vi "Correct Ascan.vi"(8 "error in":errorcluster caption="error out") -> (0 "error out":errorcluster caption="error in")   [LabVIEW 2015, in "Debug.lvlib"]
uses:
  Debug.lvlib
  Support/Filter Noise State.ctl
  <vilib>/Analysis/baseanly.llb/Mean (DBL).vi
  <vilib>/Utility/file.llb/Write Delimited Spreadsheet (DBL).vi
  <vilib>/Instr/_visa.llb/VISA Configure Serial Port (Instr).vi
  Sub VIs/DAQ/DAQ.lvlib
  Sub VIs/Digital Signal Processing/Digital Signal Processing.lvlib
  Sub VIs/Boimetry Processing/Boimetry Processing.lvlib
  <vilib>/Analysis/NI_AALBase.lvlib
  Sub VIs/Serial/Serial.lvlib
panel:
  out "进度条":u8(slide) scale=0.0..100.0
  out "DSP":dbl[](graph)
  out "Original Signal":dbl[](graph)
  in  "总长":dbl
  in  "步长":dbl
  in  "Sample Change":enum16{"1st", "2nd"}(ring)
  in  "DOUT":bool
  in  "计算":bool
  in  "采集":bool
  in  "停止按钮":bool
  out "距离点数":i32
  out "开始位置":i32
  out "状态栏":string
  # "Correct Ascan"
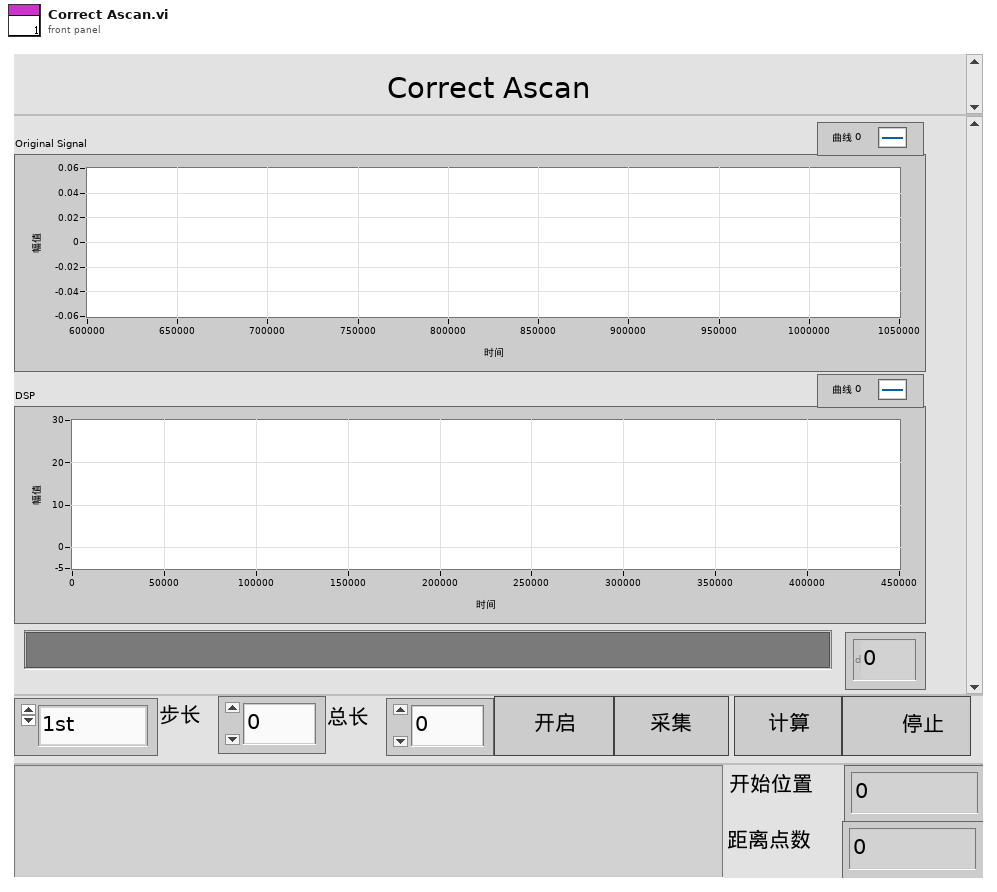
[diagram p1: front panel]
types:
  T1 = typedef "Debug.lvlib/Filter Noise State.ctl" = enum16{"Initialize", "Update Settings", "DOUT", "Sample", "Calculate", "Wait For Event", "Exit"}
  T2 = typedef "Digital Signal Processing.lvlib/DSP Configuration.ctl" = cluster{"Sampling Frequency":dbl, "filter type":T3, "RF Filter Low Frequency":dbl, "RF Filter High Frequency":dbl, "RF Filter Taps":i32, "window":T4, "RF window parameter":dbl, "filter type 2":T3, "Demodulated Filter Low Frequency":dbl, "Demodulated Filter HighFrequency":dbl, "Demodulated Filter Order":i32, "SPAN":i32, "Logarithmic Base":dbl, "Noise path":string, "Work position parameter":i32[]}
  T3 = typedef "NI_AALBase.lvlib/Filter Passband Type.ctl" = enum32{"Lowpass", "Highpass", "Bandpass", "Bandstop"}
  T4 = typedef "NI_AALPro.lvlib/windowTd.ctl" = u32
  T5 = typedef "Digital Signal Processing.lvlib/DSP Parameter.ctl" = cluster{"RF":cluster{"filter structure":enum32{"IIR 2nd Order", "IIR 4th Order"}, "Reverse Coefficients":dbl[], "Forward Coefficients":dbl[]}, "IIR Filter Cluster":cluster{"filter structure":enum32{"IIR 2nd Order", "IIR 4th Order"}, "Reverse Coefficients":dbl[], "Forward Coefficients":dbl[]}, "Noise Signal":dbl[], "SPAN":i32, "Logarithmic Base":dbl}
  T6 = cluster{"filter structure":enum32{"IIR 2nd Order", "IIR 4th Order"}, "Reverse Coefficients":dbl[], "Forward Coefficients":dbl[]}
  T7 = typedef "Boimetry Processing.lvlib/Biometry Configuration.ctl" = cluster{"Interference Width":i32, "Interference Threshold":dbl, "Cornea Len Division":i32, "Correction Data 1st Path":string, "1st_Start_Position":dbl, "Correction Data 2nd Path":string, "2nd_Start_Position":dbl, "Index Corneal":dbl, "Index Water":dbl, "Index Len":dbl, "Working Position":cluster{"FirstStart":i32, "FirstEnd":i32, "SecondStart":i32, "SecondEnd":i32}}
  T8 = cluster{"FirstStart":i32, "FirstEnd":i32, "SecondStart":i32, "SecondEnd":i32}
  T9 = typedef "DAQ.lvlib/DAQ Configuration.ctl" = cluster{"hDevice":i32, "DevNum":u8, "Configuration Parameter":i32[], "READ_MAX_LEN":i32, "DO":bool[]}
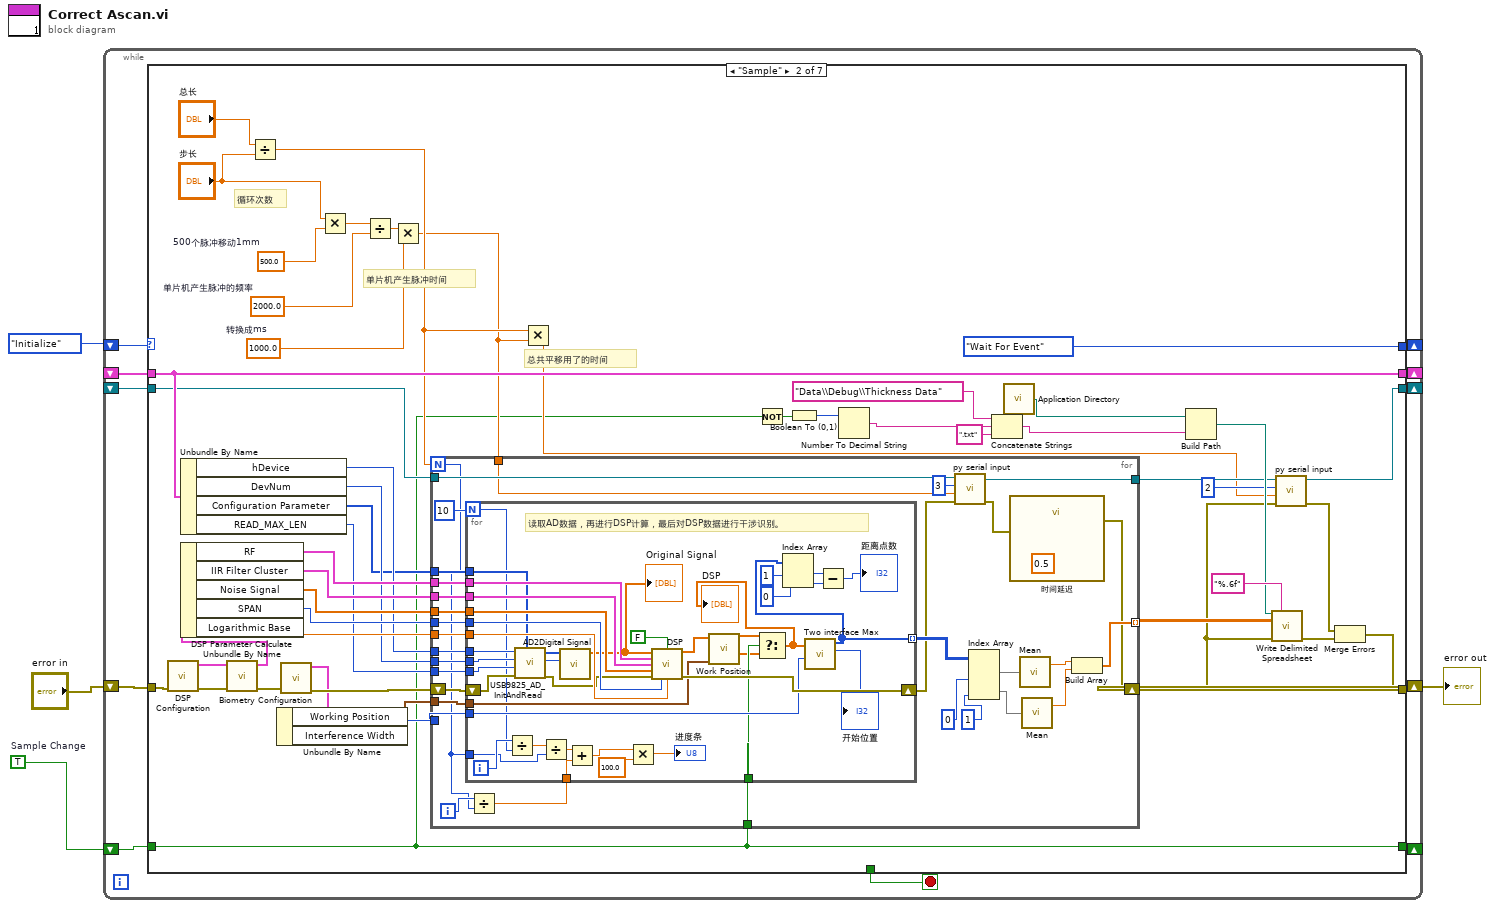
[diagram p0: block diagram]
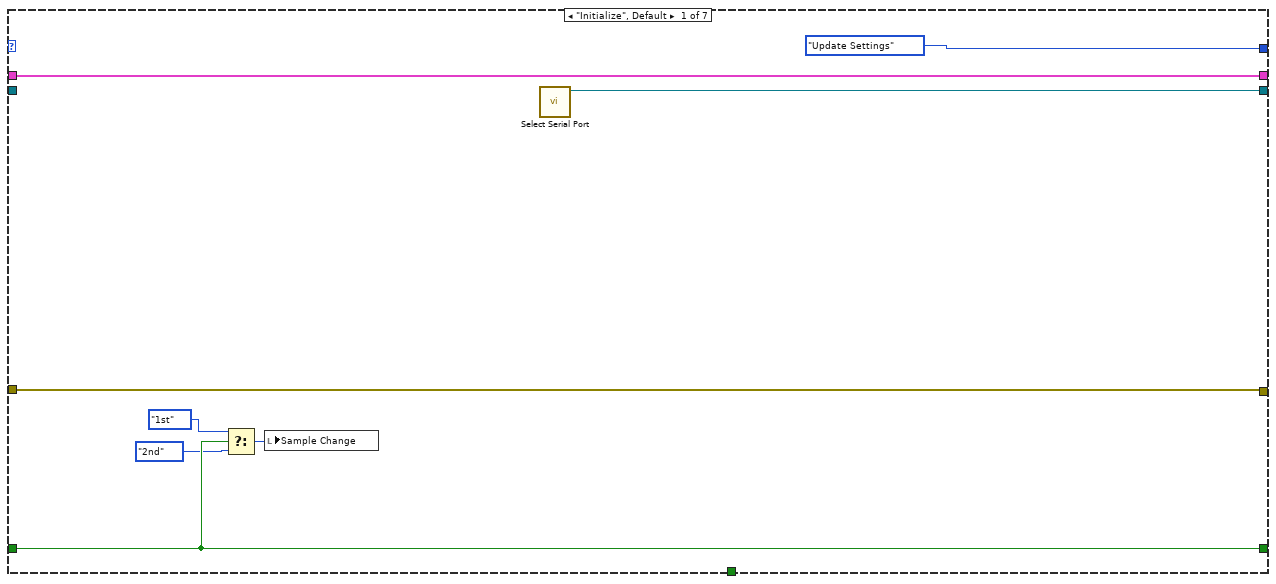
[diagram p2: hidden frame]
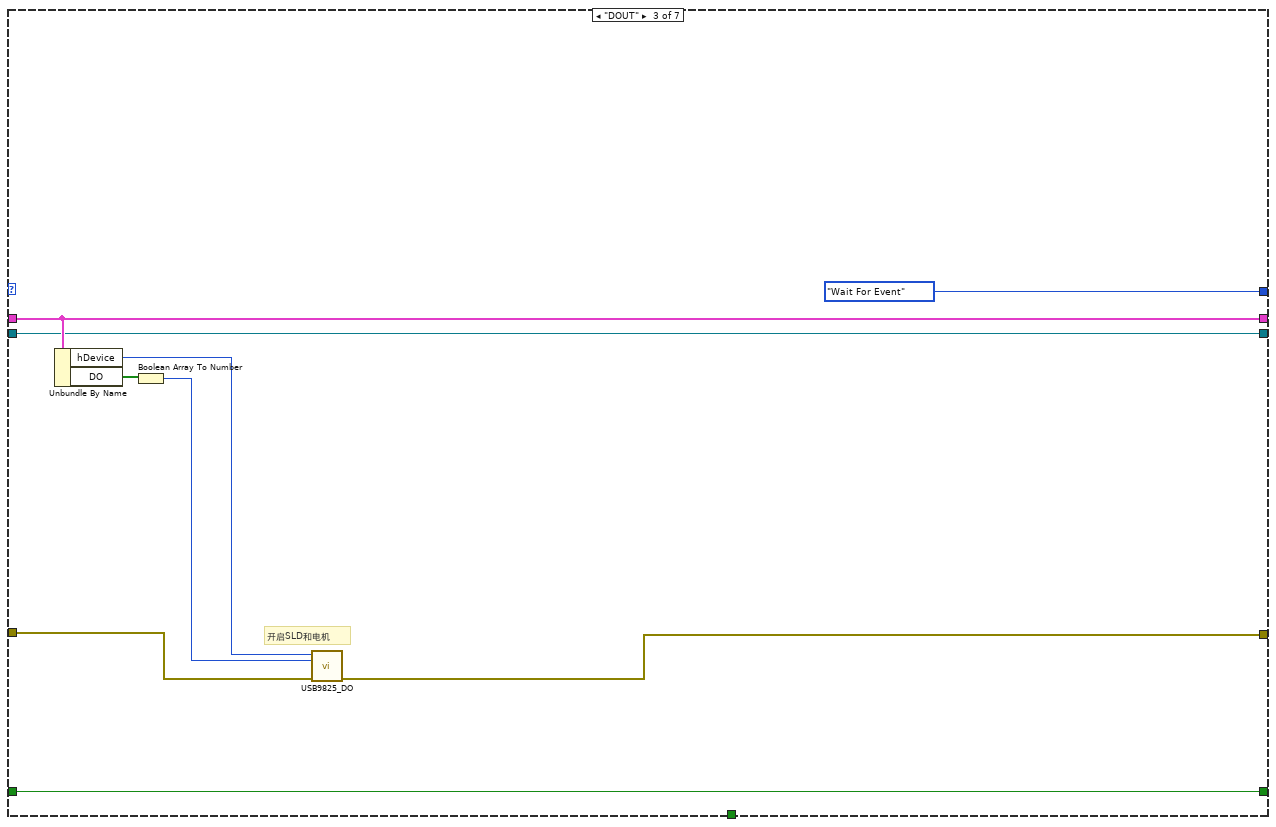
[diagram p3: hidden frame]
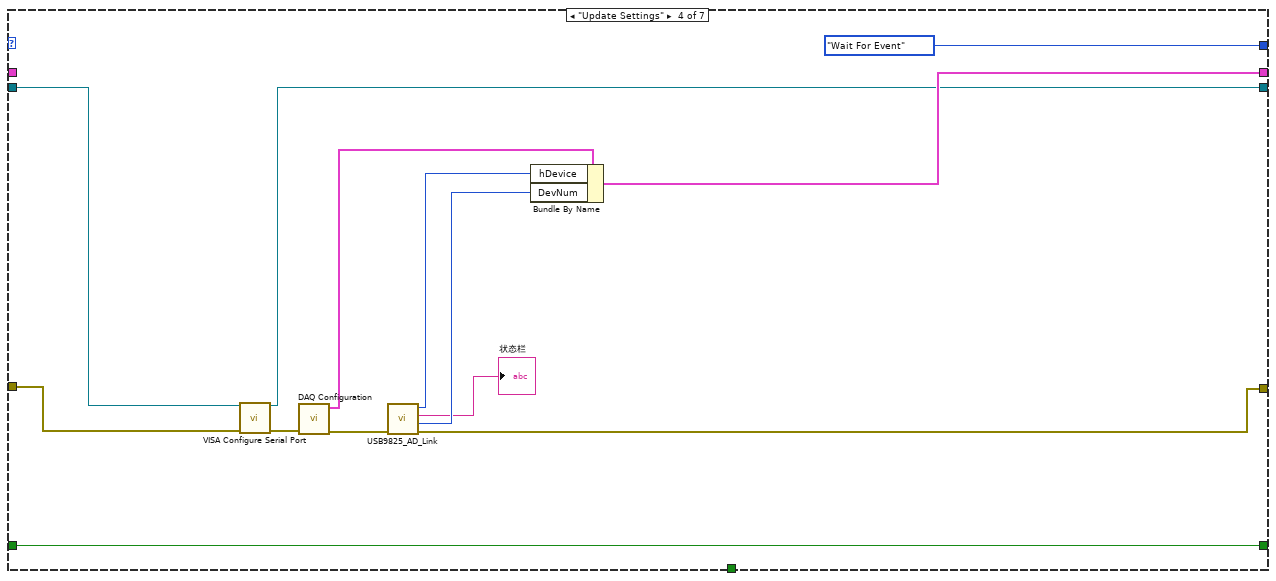
[diagram p4: hidden frame]
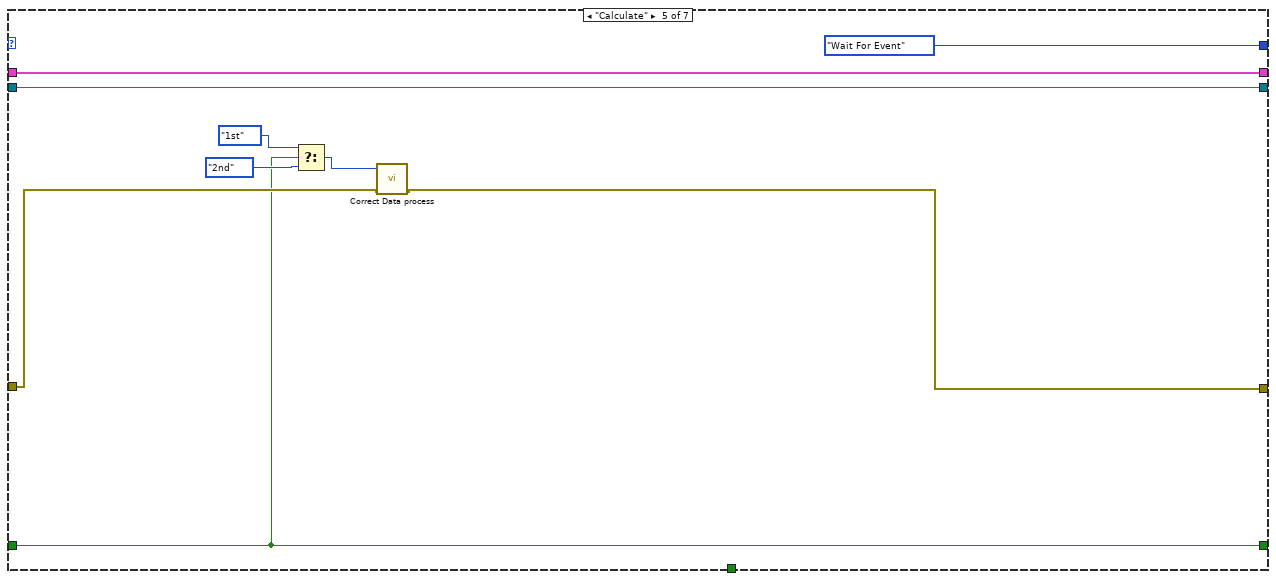
[diagram p5: hidden frame]
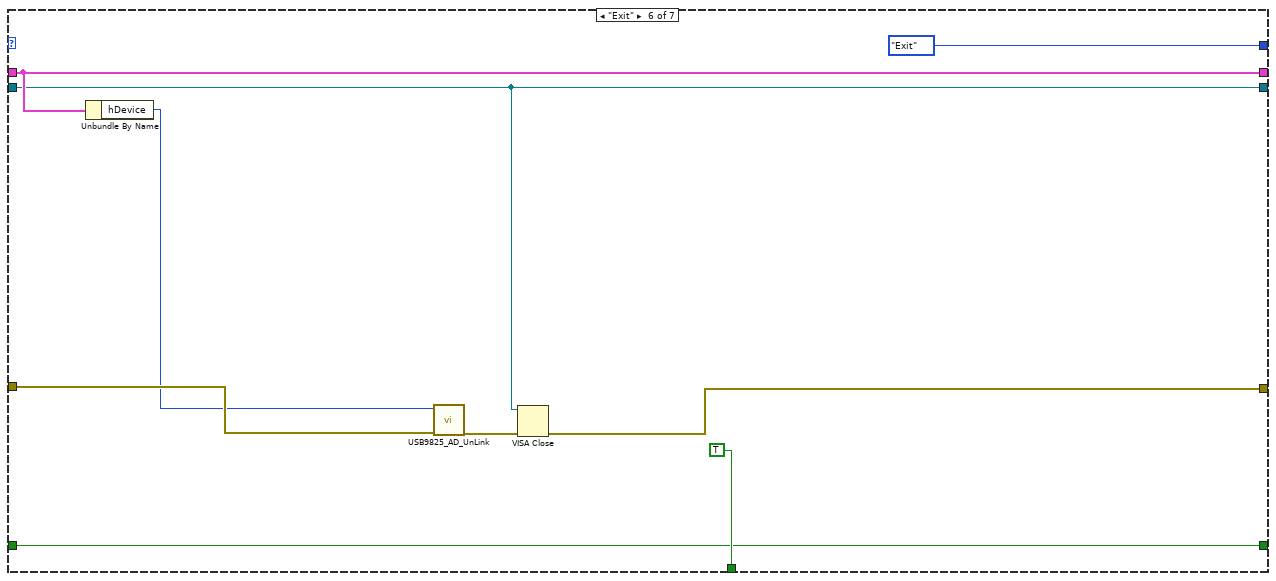
[diagram p6: hidden frame]
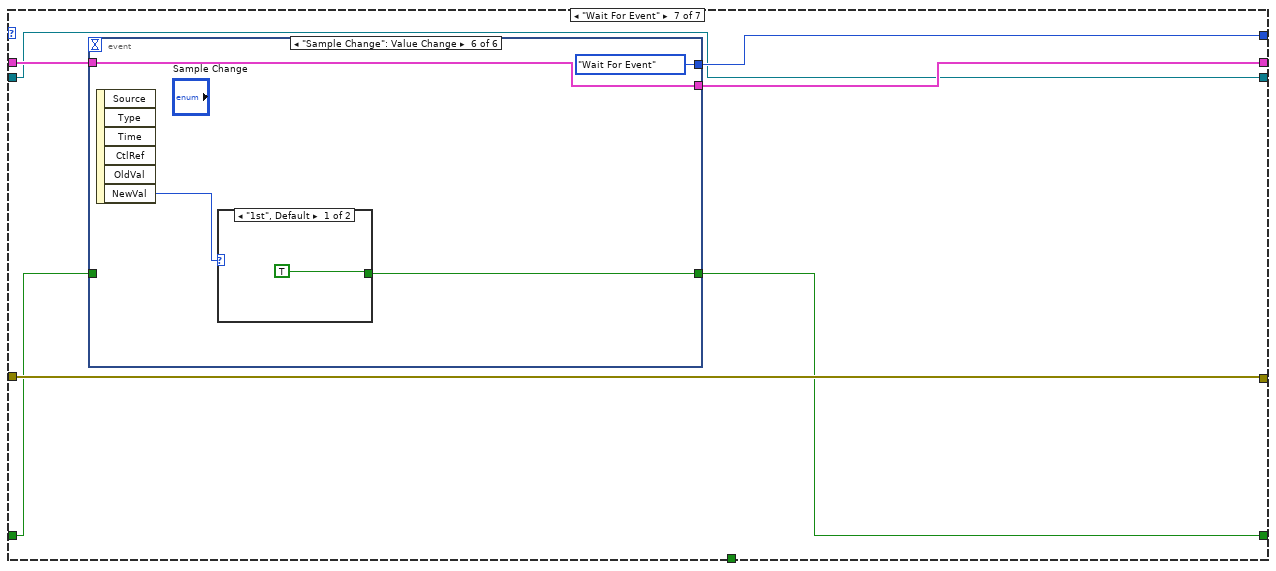
[diagram p7: hidden frame]
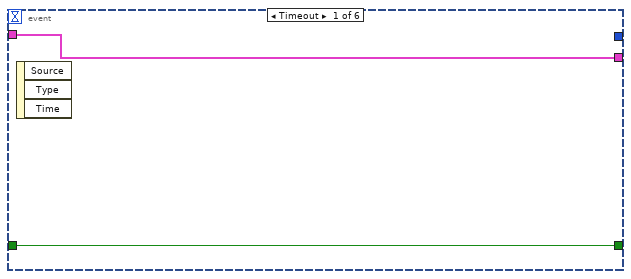
[diagram p8: hidden frame]
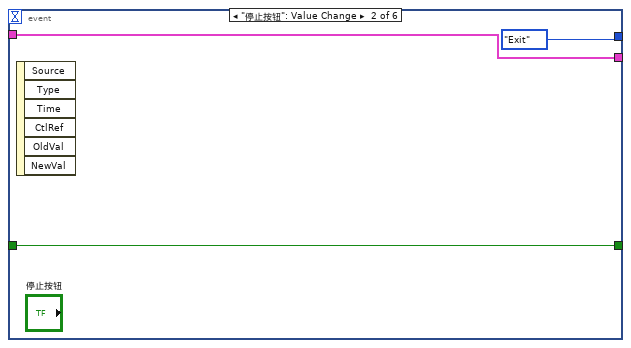
[diagram p9: hidden frame]
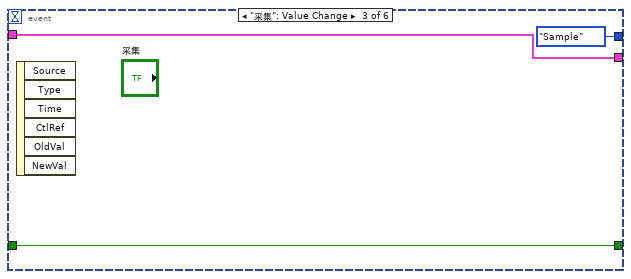
[diagram p10: hidden frame]
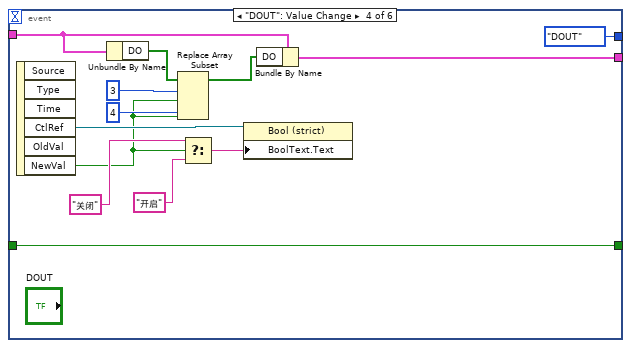
[diagram p11: hidden frame]
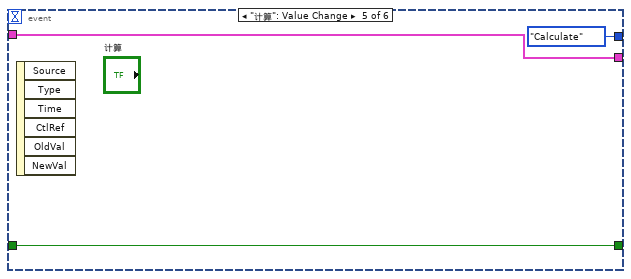
[diagram p12: hidden frame]
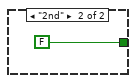
[diagram p13: hidden frame]
diagram:
  w1 = TRUE  # Sample Change
  n1 = while {
    shift-right: [w14] -> _
    shift-left: Filter_Noise_State."Initialize" ("Calculation Distance State") -> [w15]
    shift-right: [w12] -> w3
    shift-left: "error in" -> [w11]
    shift-right: [w10] -> _
    shift-left: _ -> [w9]
    shift-right: [w7] -> _
    shift-left: w1 -> [w8]
    shift-right: [w6] -> _
    shift-left: _ -> [w5]
    stop <- w13 stop-if-true
    n2 = case shown="\"Sample\"" w15 {
      tunnel: [Filter_Noise_State."Update Settings" ("Calculation Distance State") Filter_Noise_State."Wait For Event" ("Calculation Distance State") Filter_Noise_State."Wait For Event" ("Calculation Distance State") Filter_Noise_State."Wait For Event" ("Calculation Distance State") Filter_Noise_State."Wait For Event" ("Calculation Distance State") Filter_Noise_State."Exit" ("Calculation Distance State") w191] -> w14
      tunnel: [_ _ _ _ _ TRUE _] -> w13
      tunnel: w11 -> [w23 w70 w152 w155 w172 w182 w190]
      tunnel: [w23 w30 w151 w164 w171 w177 w190] -> w12
      tunnel: [w21 w71 w150 w160 w174 w181 w188] -> w10
      tunnel: w9 -> [w21 w71 w150 _ w174 w181 w189]
      tunnel: w8 -> [w19 w24 w146 w158 w167 w179 w186]
      tunnel: [w19 w24 w146 w158 w167 w179 w187] -> w7
      tunnel: [w18 w29 w145 w156 w173 w176 w185] -> w6
      tunnel: w5 -> [_ w47 w145 w157 w173 w176 w185]
      frame "Initialize", Default {
        n3 = Select(t=enum16{"1st", "2nd"}."1st" ("f"), s=w19, f=enum16{"1st", "2nd"}."2nd" ("Sample Change")) -> (s? t:f=w20:enum16{"1st", "2nd"})
        n4 = local write "Sample Change"(w20) -> ()
        n5 = call "Select Serial Port.vi"() -> ("VISA资源名称 2"=w18:refnum<visa-resource-name>)  [unwired: 11 in]
      }
      frame "Sample" {
        w27 = 1000.0  # 转换成ms
        w38 = 2000.0  # 单片机产生脉冲的频率
        w40 = 500.0  # 500个脉冲移动1mm
        # "总共平移用了的时间"
        # "单片机产生脉冲时间"
        # "循环次数"
        n6 = call "DSP Configuration.vi"("error in (no error)"=w70) -> ("error out"=w69:errorcluster, "DSP Parameter Output"=w62:T2)  [unwired: 9 in]
        n7 = Unbundle By Name(w71) -> ("hDevice"=w46:i32, "DevNum"=w45:u8, "Configuration Parameter"=w43:i32[], "READ_MAX_LEN"=w44:i32)
        n8 = call "DSP Parameter Calculate.vi"("error in (no error)"=w69, "DSP Configuration"=w62) -> ("error out"=w61:errorcluster, "DSP Parameter"=w68:T5)  [unwired: 8 in]
        n9 = Unbundle By Name(w68) -> ("RF"=w67:T6, "IIR Filter Cluster"=w66:T6, "Noise Signal"=w63:dbl[], "SPAN"=w65:i32, "Logarithmic Base"=w64:dbl)
        n10 = Divide(x="总长", y="步长") -> (x/y=w34:dbl)
        n11 = call "Biometry Configuration.vi"("error in (no error)"=w61) -> ("error out"=w60:errorcluster, "Biometry Configuration"=w59:T7)  [unwired: 9 in]
        n12 = Unbundle By Name(w59) -> ("Working Position"=w58:T8, "Interference Width"=w57:i32)
        n13 = Multiply(x="步长", y=w40) -> (x*y=w39:dbl)
        n14 = Divide(x=w39, y=w38) -> (x/y=w28:dbl)
        n15 = Multiply(x=w28, y=w27) -> (x*y=w26:dbl)
        n16 = for {
          N: w34 -> [w74]
          tunnel: w67 -> [w105]
          tunnel: w66 -> [w104]
          tunnel: w65 -> [w103]
          tunnel: w64 -> [w102]
          tunnel: w63 -> [w100]
          tunnel: w58 -> [w98]
          tunnel: w57 -> [w97]
          tunnel: w24 -> [w96]
          shift-right: [w77] -> w35
          shift-left: w60 -> [w99]
          tunnel: [w88] -> w56 mode=indexing
          tunnel: w47 -> [w86]
          tunnel: w46 -> [w85]
          tunnel: w45 -> [w84]
          tunnel: w44 -> [w83]
          tunnel: w43 -> [w82]
          tunnel: w26 -> [w81]
          tunnel: [w79] -> w37
          i -> [w75]
          n17 = Divide(x=w75, y=w74) -> (x/y=w73:dbl)
          n18 = for {
            N: 10 -> [w116]
            shift-right: [w144] -> w87
            shift-left: w99 -> [w139]
            tunnel: w105 -> [w143]
            tunnel: w104 -> [w142]
            tunnel: w103 -> [w141]
            tunnel: w102 -> [w140]
            tunnel: w100 -> [w135]
            tunnel: w98 -> [w132]
            tunnel: w97 -> [w131]
            tunnel: w96 -> [w130]
            tunnel: [w124] -> w95 mode=indexing
            tunnel: w85 -> [w129]
            tunnel: w84 -> [w128]
            tunnel: w83 -> [w127]
            tunnel: w82 -> [w126]
            tunnel: w74 -> [w114]
            tunnel: w73 -> [w111]
            i -> [w117]
            # "读取AD数据，再进行DSP计算，最后对DSP数据进行干涉识别。"
            n19 = Divide(x=w117, y=w116) -> (x/y=w115:dbl)
            n20 = call "USB9825_AD_InitAndRead.vi"("Configuration Parameter"=w126, "错误输入（无错误）"=w139, "READ_MAX_LEN"=w127, "DevNum"=w128, "hDevice"=w129) -> ("错误输出"=w136:errorcluster, "通道数"=w137:i32, "AD"=w138:i16[])  [unwired: 3 in, 1 out]
            n21 = Divide(x=w115, y=w114) -> (x/y=w112:dbl)
            n22 = call "AD2Digital Signal.vi"("通道数"=w137, "AD"=w138) -> ("CH1"=w133:dbl[])  [unwired: 8 in, 1 out]
            "Original Signal" <- w133
            n23 = Add(x=w112, y=w111) -> (x+y=w110:dbl)
            n24 = Multiply(x=w110, y=100.0) -> (x*y=→"进度条":dbl)
            n25 = call "DSP.vi"("Input Signal"=w133, "Minus Noise(F : Don't)"=FALSE ("Smooth(F : Don't)"), "RF"=w143, "IIR Filter Cluster"=w142, "Noise Signal"=w135, "error in (no error)"=w136, "SPAN"=w141, "Logarithmic Base"=w140) -> ("DSP signal"=w118:dbl[], "error out"=w144:errorcluster)  [unwired: 6 in]
            n26 = call "Work Position.vi"("Working Position"=w132, "S"=w118) -> ("S_2nd_part"=w106:dbl[], "S_1st_part"=w107:dbl[])  [unwired: 4 in, 4 out]
            n27 = Select(t=w107, s=w130, f=w106) -> (s? t:f=w108:dbl[])
            "DSP" <- w108
            n28 = call "Two interface Max.vi"("Width"=w131, "S"=w108) -> ("MAX_Index"=→"开始位置":i32, "INDEX"=w124:i32[])  [unwired: 8 in]
            n29 = Index Array(array=w124, index #1=1 ("索引"), index #2=0 ("索引")) -> (element #1=w120:i32, element #2=w121:i32)
            n30 = Subtract(x=w120, y=w121) -> (x-y=→"距离点数":i32)
          }
          n31 = call "py serial input.vi"("错误输入（无错误）"=w87, "parameter"=w81, "item"=u8 3, "VISA资源名称"=w86) -> ("错误输出"=w78:errorcluster, "VISA资源名称输出"=w79:refnum<visa-resource-name>)  [unwired: 6 in]
          n32 = Index Array(array=w95, index (col) #1=0 ("禁用的索引 (列)"), index (col) #2=1 ("索引 (列)")) -> (element #1=w92:i32[], element #2=w91:i32[])  [unwired: 2 in]
          n33 = call "时间延迟"("error in (no error)"=w78, "Delay Time (s)"=0.5) -> ("error out"=w77:errorcluster)  [unwired: 9 in]
          n34 = call-poly <vilib>:"Mean.vi"("X"=w92) -> ("mean"=w89:dbl)  [unwired: 1 out]
          n35 = call-poly <vilib>:"Mean.vi"("X"=w91) -> ("mean"=w90:dbl)  [unwired: 1 out]
          n36 = Build Array(w89, w90) -> (w88:dbl[])
        }
        n37 = Multiply(x=w34, y=w26) -> (x*y=w33:dbl)
        n38 = Not(x=w24) -> (.not. x?=w25:bool)
        n39 = Boolean To (0,1)(Boolean=w25) -> (0, 1=w52:i16)
        n40 = Number To Decimal String(number=w52) -> (decimal integer string=w51:string)  [unwired: 1 in]
        n41 = Concatenate Strings("Data\\Debug\\Thickness Data" ("字符串"), w51, ".txt" ("字符串")) -> (w49:string)
        n42 = call <vilib>:"Application Directory.vi"() -> ("Application Directory"=w54:path)
        n43 = Build Path(base path=w54, name or relative path=w49) -> (appended path=w48:path)
        n44 = call-poly <vilib>:"Write Delimited Spreadsheet.vi"("file path (dialog if empty)"=w48, "format (%.3f)"="%.6f", "2D data"=w56, "error in (no error)"=w35) -> ("error out"=w32:errorcluster)  [unwired: 10 in, 1 out]
        n45 = call "py serial input.vi"("错误输入（无错误）"=w35, "parameter"=w33, "item"=u8 2, "VISA资源名称"=w37) -> ("错误输出"=w31:errorcluster, "VISA资源名称输出"=w29:refnum<visa-resource-name>)  [unwired: 6 in]
        n46 = Merge Errors(w31, w32) -> (w30:errorcluster)
      }
      frame "DOUT" {
        # "开启SLD和电机"
        n47 = Unbundle By Name(w150) -> ("hDevice"=w149:i32, "DO"=w148:bool[])
        n48 = Boolean Array To Number(Boolean array=w148) -> (number=w147:u32)
        n49 = call "USB9825_DO.vi"("Error In"=w152, "pDO"=w147, "hDevice"=w149) -> ("Error Out"=w151:errorcluster)  [unwired: 8 in]
      }
      frame "Update Settings" {
        n50 = call-poly "VISA Configure Serial Port"("VISA resource name"=w157, "error in (no error)"=w155) -> ("VISA resource name out"=w156:refnum<visa-resource-name>, "error out"=w154:errorcluster)  [unwired: 12 in]
        n51 = call "DAQ Configuration.vi"("error in (no error)"=w154) -> ("error out"=w165:errorcluster, "parameter output"=w163:T9)  [unwired: 9 in]
        n52 = call "USB9825_AD_Link.vi"("Error In"=w165) -> ("Error Out"=w164:errorcluster, "DevNum"=w161:i32, "设备属性"=→"状态栏":string, "hDevice"=w162:i32)  [unwired: 7 in]
        n53 = Bundle By Name(cluster=w163, "hDevice"=w162, "DevNum"=w161) -> (w160:T9)
      }
      frame "Calculate" {
        n54 = Select(t=enum16{"1st", "2nd"}."1st" ("f"), s=w167, f=enum16{"1st", "2nd"}."2nd" ("Sample Change")) -> (s? t:f=w168:enum16{"1st", "2nd"})
        n55 = call "Correct Data process.vi"("error in"=w172, "区域选择"=w168) -> ("error out"=w171:errorcluster)  [unwired: 9 in]
      }
      frame "Exit" {
        n56 = Unbundle By Name(w181) -> ("hDevice"=w180:i32)
        n57 = call "USB9825_AD_UnLink.vi"("Error In"=w182, "hDevice"=w180) -> ("Error Out"=w178:errorcluster)  [unwired: 9 in]
        n58 = VISA Close(VISA resource name=w176, error in (no error)=w178) -> (error out=w177:errorcluster)
      }
      frame "Wait For Event" {
        n59 = event shown="[5] \"Sample Change\": Value Change" {
          selector: _ -> [_ _ _ _ _ _]
          dyn-events: _ -> [_ _ _ _ _ _]
          timeout: _ -> [_ _ _ _ _ _]
          tunnel: [_ Filter_Noise_State."Exit" ("Calculation Distance State") Filter_Noise_State."Sample" ("Calculation Distance State") Filter_Noise_State."DOUT" ("Calculation Distance State") Filter_Noise_State."Calculate" ("Calculation Distance State") Filter_Noise_State."Wait For Event" ("Calculation Distance State")] -> w191
          tunnel: w189 -> [w193 w195 w198 w203 w214 w216]
          tunnel: [w193 w195 w198 w201 w214 w216] -> w188
          tunnel: [w192 w194 w197 w200 w213 w217] -> w187
          tunnel: w186 -> [w192 w194 w197 w200 w213 _]
          event Timeout {
            n60 = event-data() -> ()  [unwired: 1 in, 3 out]
          }
          event "停止按钮": Value Change {
            n61 = event-data() -> ()  [unwired: 1 in, 6 out]
          }
          event "采集": Value Change {
            n62 = event-data() -> ()  [unwired: 1 in, 6 out]
          }
          event "DOUT": Value Change {
            n63 = event-data() -> ("CtlRef"=w211:refnum<vi>, "NewVal"=w204:bool)  [unwired: 1 in, 4 out]
            n64 = Unbundle By Name(w203) -> ("DO"=w207:bool[])
            n65 = Replace Array Subset(array=w207, new element #1=w204, index #1=3 ("索引"), new element #2=w204, index #2=4 ("索引")) -> (w202:bool[])
            n66 = Select(t="关闭", s=w204, f="开启") -> (s? t:f=w210:string)
            n67 = property class="Bool (strict)"(reference=w211, "BoolText.Text"=w210) -> ()  [unwired: 1 in, 2 out]
            n68 = Bundle By Name(cluster=w203, "DO"=w202) -> (w201:T9)
          }
          event "计算": Value Change {
            n69 = event-data() -> ()  [unwired: 1 in, 6 out]
          }
          event "Sample Change": Value Change {
            n70 = event-data() -> ("NewVal"=w218:enum16{"1st", "2nd"})  [unwired: 1 in, 5 out]
            n71 = case shown="\"1st\", Default" w218 {
              tunnel: [TRUE FALSE] -> w217
              frame "1st", Default {
              }
              frame "2nd" {
              }
            }
          }
        }
      }
    }
  }
  "error out" <- w3
